vi "Create_Default_DistParts.vi"(8 "error in (no error)":errorcluster, 11 "IB_MSI in":refnum<class "IB_MSI.lvclass">) -> (0 "error out":errorcluster, 3 "IB_MSI out":refnum<class "IB_MSI.lvclass">)   [LabVIEW 2020, in "IB_MSI.lvclass"]
uses:
  <vilib>/AppBuilder/IB_Classes/MSI/IB_MSI.lvclass
  <vilib>/AppBuilder/IB_Classes/MSI/IB_MSI.lvclass/IB_MSI.ctl
  <resource>/Framework/Providers/Builds/Installer/CDK_sTypeDef_FindProduct.ctl
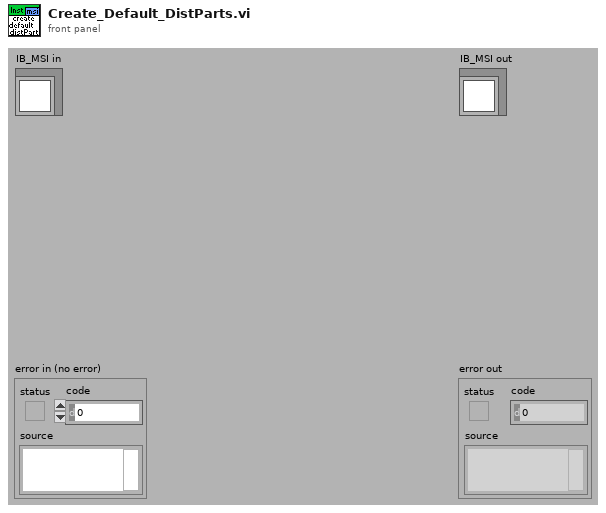
[diagram p1: front panel]
types:
  T1 = typedef "CDK_sTypeDef_FindProduct.ctl" = enum16{"LabVIEW RTE", "DataSocket", "USI", "CVI RTE", "LVDeployableLic"}
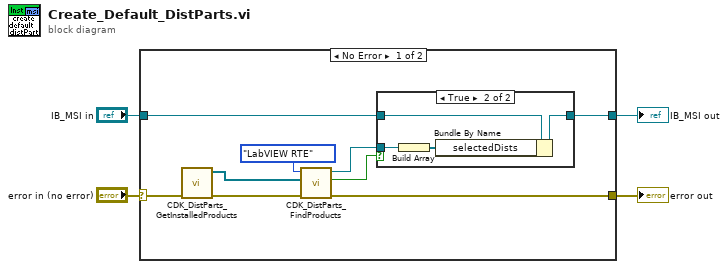
[diagram p0: block diagram]
diagram:
  n1 = case shown="No Error" "error in (no error)" {
    selector: "error in (no error)" -> [w12 w20]
    tunnel: [w8 w20] -> w3
    tunnel: [w13 w19] -> w1
    tunnel: "IB_MSI in" -> [w7 w19]
    frame No Error {
      n2 = call <resource>:"CDK_DistParts_GetInstalledProducts.vi"("ErrIn"=w12) -> ("ErrOut"=w9:errorcluster, "installed products"=w6:refnum<class "IB_DistPart.lvclass">[])  [unwired: 9 in]
      n3 = call <resource>:"CDK_DistParts_FindProducts.vi"("ErrIn"=w9, "InstalledProducts"=w6, "ProductName"=CDK_sTypeDef_FindProduct."LabVIEW RTE") -> ("ErrOut"=w8:errorcluster, "Found?"=w10:bool, "RunTime Engine"=w5:refnum<class "IB_DistPart.lvclass">)  [unwired: 5 in, 1 out]
      n4 = case shown="True" w10 {
        tunnel: [w14 w18] -> w13
        tunnel: w7 -> [w14 w16]
        tunnel: w5 -> [_ w15]
        frame False {
        }
        frame True {
          n5 = Build Array(w15) -> (w17:refnum<class "IB_DistPart.lvclass">[])
          n6 = Bundle By Name(cluster=w16, "selectedDists"=w17) -> (w18:refnum<class "IB_MSI.lvclass">)
        }
      }
    }
    frame Error {
    }
  }
  "error out" <- w3
  "IB_MSI out" <- w1
